vi "To and From String Array Test.vi"() -> ()   [LabVIEW 2015, in "Parallel Steps Tests.lvlib"]
uses:
  Parallel Steps Tests.lvlib
  Config/Parallel Step Config.lvclass
  classes/Step/Config/Step Config.lvclass
panel:
  out "Step String Array 2":string[](array[string])
  out "Step String Array":string[](array[string])
  out "Pass":bool
  out "error out":errorcluster
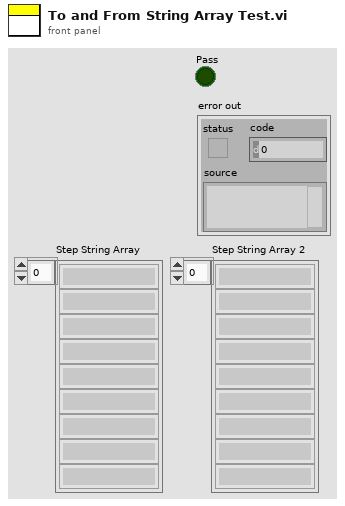
[diagram p1: front panel]
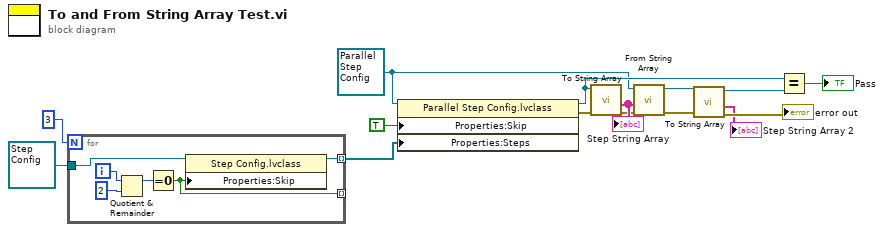
[diagram p0: block diagram]
diagram:
  w9 = refnum<class "Parallel Step Config.lvclass"> refnum ("Parallel Step Config.lvclass")
  n1 = for {
    N: 3 -> [_]
    tunnel: refnum<class "Step Config.lvclass"> refnum ("Step Config.lvclass") -> [w21]
    tunnel: [w17] -> _ mode=indexing
    tunnel: [w16] -> w6 mode=indexing
    i -> [w20]
    n2 = Quotient & Remainder(x=w20, y=2) -> (x-y*floor(x/y)=w18:i32)  [unwired: 1 out]
    n3 = Equal To 0?(x=w18) -> (x = 0?=w17:bool)
    n4 = property class="Step Config.lvclass"(reference=w21, "Properties:Skip"=w17) -> (reference out=w16:refnum<class "Step Config.lvclass">)  [unwired: 1 in, 1 out]
  }
  n5 = property class="Parallel Step Config.lvclass"(reference=w9, "Properties:Skip"=TRUE, "Properties:Steps"=w6) -> (reference out=w13:refnum<class "Parallel Step Config.lvclass">, error out=w10:errorcluster)  [unwired: 1 in]
  n6 = call-dynamic "To String Array.vi"("error in (no error)"=w10, "Parallel Step Config in"=w13) -> ("error out"=w12:errorcluster, "Step String Array"=w15:string[])  [unwired: 7 in, 1 out]
  "Step String Array" <- w15
  n7 = call-dynamic "From String Array.vi"("error in (no error)"=w12, "String Array"=w15, "Parallel Step Config in"=w9) -> ("error out"=w5:errorcluster, "Parallel Step Config out"=w4:refnum<class "Parallel Step Config.lvclass">)  [unwired: 6 in, 1 out]
  n8 = call-dynamic "To String Array.vi"("error in (no error)"=w5, "Parallel Step Config in"=w4) -> ("error out"=→"error out":errorcluster, "Step String Array"=→"Step String Array 2":string[], "Parallel Step Config out"=w3:refnum<class "Parallel Step Config.lvclass">)  [unwired: 7 in]
  n9 = Equal?(x=w13, y=w3) -> (x = y?=→"Pass":bool)
